vi "ThreadCfg - Write TxPkt Config.vi"(8 "error in (no error)":errorcluster, 10 "threadOptions":T1 {"pclDecimation" max=16 step=1; "loopPeriod" max=16 step=1; "targetPriority" min=-2 max=16 step=1; "targetProcessor" min=-2 max=16 step=1}, 11 "Node Ptr In":T4 format="%.0x") -> (0 "error out":errorcluster, 3 "Node Ptr Out":T4 format="%.0x")   [LabVIEW 2016, in "UDP-Custom-Device System Explorer.lvlib"]
uses:
  UDP-Custom-Device System Explorer.lvlib
  <vilib>/NI Veristand/Custom Device API/Custom Device Item Ref.ctl
  Types/Threading/Thread Configuration.ctl
  Types/Threading/Thread Sync Reference.ctl
  Shared/Types/Shared - Thread Management.ctl
  Property Accessors/Tx Packet Accessors.lvlib
  Property Accessors/Shared Packet Accessors.lvlib
  <vilib>/NI VeriStand/Custom Device API/Custom Device API.lvlib
  Shared/UDP-Custom-Device Shared.lvlib
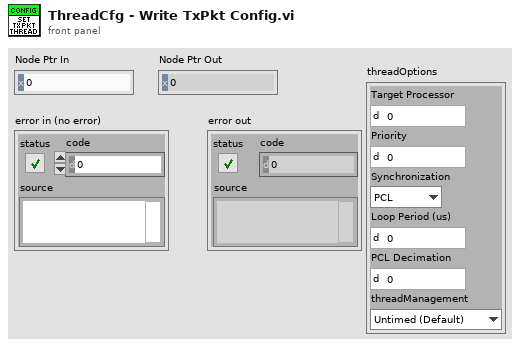
[diagram p1: front panel]
types:
  T1 = typedef "UDP-Custom-Device System Explorer.lvlib/Thread Configuration.ctl" = cluster{"targetProcessor":i8, "targetPriority":i16, "Synchronization":T2, "loopPeriod":u32, "pclDecimation":u16, "threadManagement":T3}
  T2 = typedef "UDP-Custom-Device System Explorer.lvlib/Thread Sync Reference.ctl" = enum16{"PCL", "Async"}
  T3 = typedef "UDP-Custom-Device Shared.lvlib/Shared - Thread Management.ctl" = enum16{"Untimed (Default)", "Timed (High Priority)"}
  T4 = typedef "Custom Device API.lvlib/Custom Device Item Ref.ctl" = u64
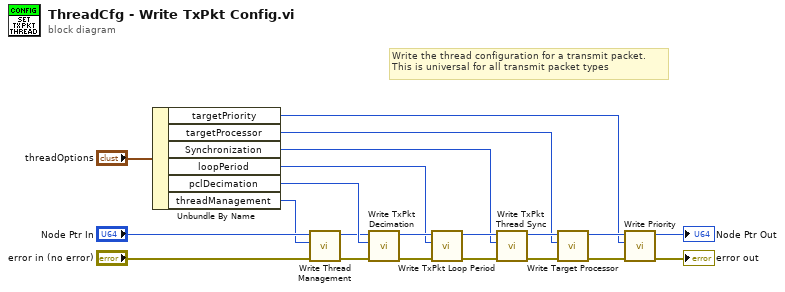
[diagram p0: block diagram]
diagram:
  # "Write the thread configuration for a transmit packet.\nThis is universal for all transmit packet types"
  n1 = Unbundle By Name("threadOptions") -> ("targetPriority"=w6:i16, "targetProcessor"=w7:i8, "Synchronization"=w8:T2, "loopPeriod"=w9:u32, "pclDecimation"=w10:u16, "threadManagement"=w1:T3)
  n2 = call "Write Thread Management.vi"("error in (no error)"="error in (no error)", "Thread Management"=w1, "Node Ptr"="Node Ptr In") -> ("error out"=w2:errorcluster, "Node Ptr out"=w4:T4)  [unwired: 7 in]
  n3 = call "Write TxPkt Decimation.vi"("error in (no error)"=w2, "Decimation"=w10, "Node Ptr"=w4) -> ("error out"=w21:errorcluster, "Node Ptr out"=w14:T4)  [unwired: 7 in]
  n4 = call "Write TxPkt Loop Period.vi"("error in (no error)"=w21, "loopPeriod"=w9, "Node Ptr"=w14) -> ("error out"=w20:errorcluster, "Node Ptr out"=w13:T4)  [unwired: 7 in]
  n5 = call "Write TxPkt Thread Sync.vi"("error in (no error)"=w20, "threadSync"=w8, "Node Ptr"=w13) -> ("error out"=w19:errorcluster, "Node Ptr out"=w12:T4)  [unwired: 7 in]
  n6 = call "Write Target Processor.vi"("error in (no error)"=w19, "targetProcessor"=w7, "Node Ptr"=w12) -> ("error out"=w18:errorcluster, "Node Ptr out"=w11:T4)  [unwired: 7 in]
  n7 = call "Write Priority.vi"("error in (no error)"=w18, "targetPriority"=w6, "Node Ptr"=w11) -> ("error out"=→"error out":errorcluster, "Node Ptr out"=→"Node Ptr Out":T4)  [unwired: 7 in]
